vi "Labview Sender Client#2.vi"() -> ()   [LabVIEW 2020]
panel:
  out "Random Array":dbl[](array[numeric])
  out "mode (standard)":T1(ring)
  out "output cluster":T2
  in  "stop":bool
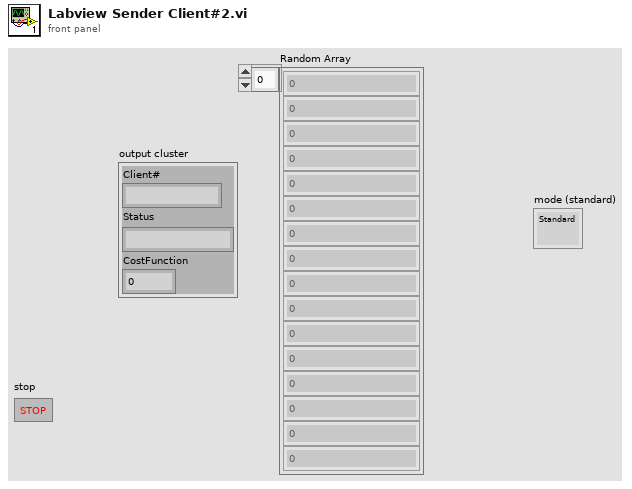
[diagram p1: front panel]
types:
  T1 = enum16{"Standard", "Buffered", "CRLF", "Immediate"}
  T2 = cluster{"Client#":string, "Status":string, "CostFunction":dbl}
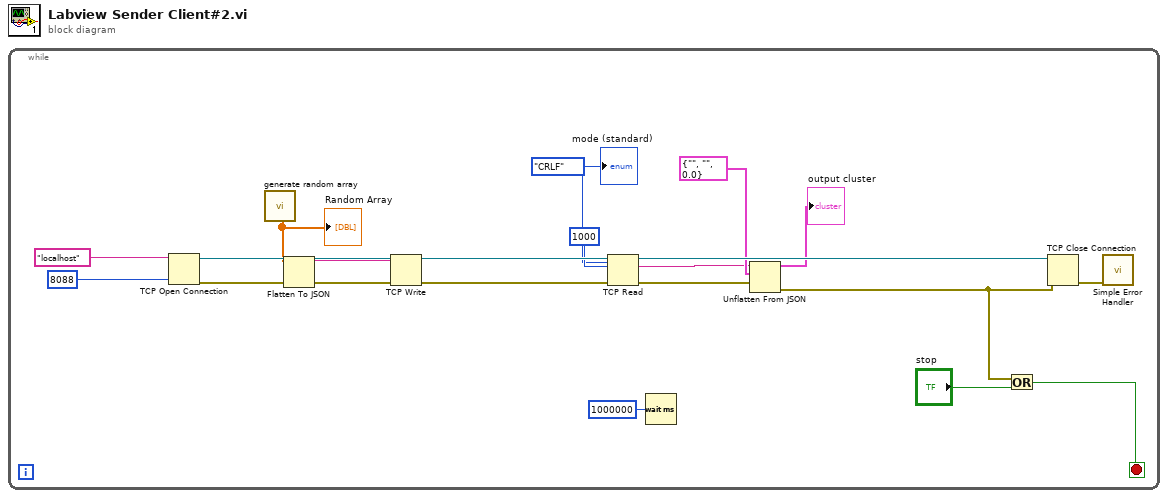
[diagram p0: block diagram]
diagram:
  n1 = while {
    stop <- w11 stop-if-true
    w8 = T1."CRLF" ("mode (standard)")
    n2 = TCP Open Connection(address="localhost", remote port or service name=8088) -> (connection ID=w20:refnum<k5>, error out=w19:errorcluster)  [unwired: 3 in]
    n3 = call "generate random array.vi"() -> ("Random Array"=w3:dbl[])  [unwired: 11 in]
    "Random Array" <- w3
    n4 = Flatten To JSON(anything=w3, error in (no error)=w19) -> (JSON string=w15:string, 11:w16:errorcluster)  [unwired: 1 in]
    n5 = TCP Write(connection ID=w20, data in=w15, error in (no error)=w16) -> (connection ID out=w14:refnum<k5>, error out=w13:errorcluster)  [unwired: 1 in, 1 out]
    n6 = TCP Read(connection ID=w14, bytes to read=1000, error in (no error)=w13, 7:w8) -> (connection ID out=w5:refnum<k5>, data out=w1:string, error out=w7:errorcluster)  [unwired: 1 in]
    n7 = Wait (ms)(milliseconds to wait=u32 1000000) -> ()  [unwired: 1 out]
    n8 = Unflatten From JSON(JSON string=w1, type and defaults=T2 {"Client#"="", "Status"="", "CostFunction"=0.0} ("cluster"), error in (no error)=w7) -> (value=→"output cluster":T2, error out=w6:errorcluster)  [unwired: 4 in]
    n9 = Or(x=w6, y="stop") -> (x .or. y?=w11:bool)
    n10 = TCP Close Connection(connection ID=w5, error in (no error)=w6) -> (error out=w18:errorcluster)  [unwired: 1 in, 1 out]
    n11 = call <vilib>:"Simple Error Handler.vi"("error in (no error)"=w18) -> ()  [unwired: 4 in, 5 out]
    "mode (standard)" <- w8
  }
